vi "DMM_Main.vi"() -> ()   [LabVIEW 2014]
panel:
  out "NumRef":refnum<data-value>
  out "SignalsRef":refnum<data-value>
  in  "Start Process":bool
  in  "Exit Program":bool
  in  "Halt Measuring":bool
  out "Baseline Reference":dbl
  out "Measuring Signals":dbl[](graph)
  in  "Pick Baseline Ref":bool
  out "SampleNum":i32
  out "State":string
  in  "Comments":string
  in  "File Path":path
  in  "Sampling Rate (point / sec)":u32
  in  "Measurement":enum16{"Resistance", "Current"}(ring)
  in  "Baseline Pick":enum16{"Manual", "Auto"}(ring)
  in  "DMM7510 COM":refnum<visa-resource-name>
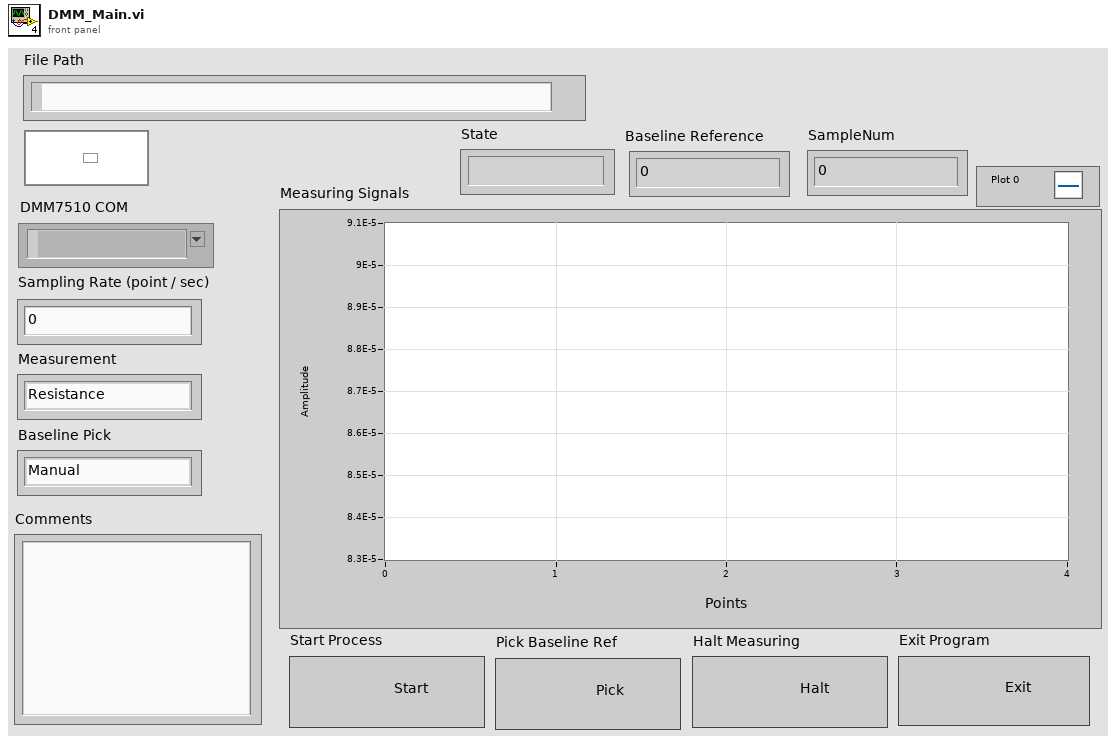
[diagram p1: front panel]
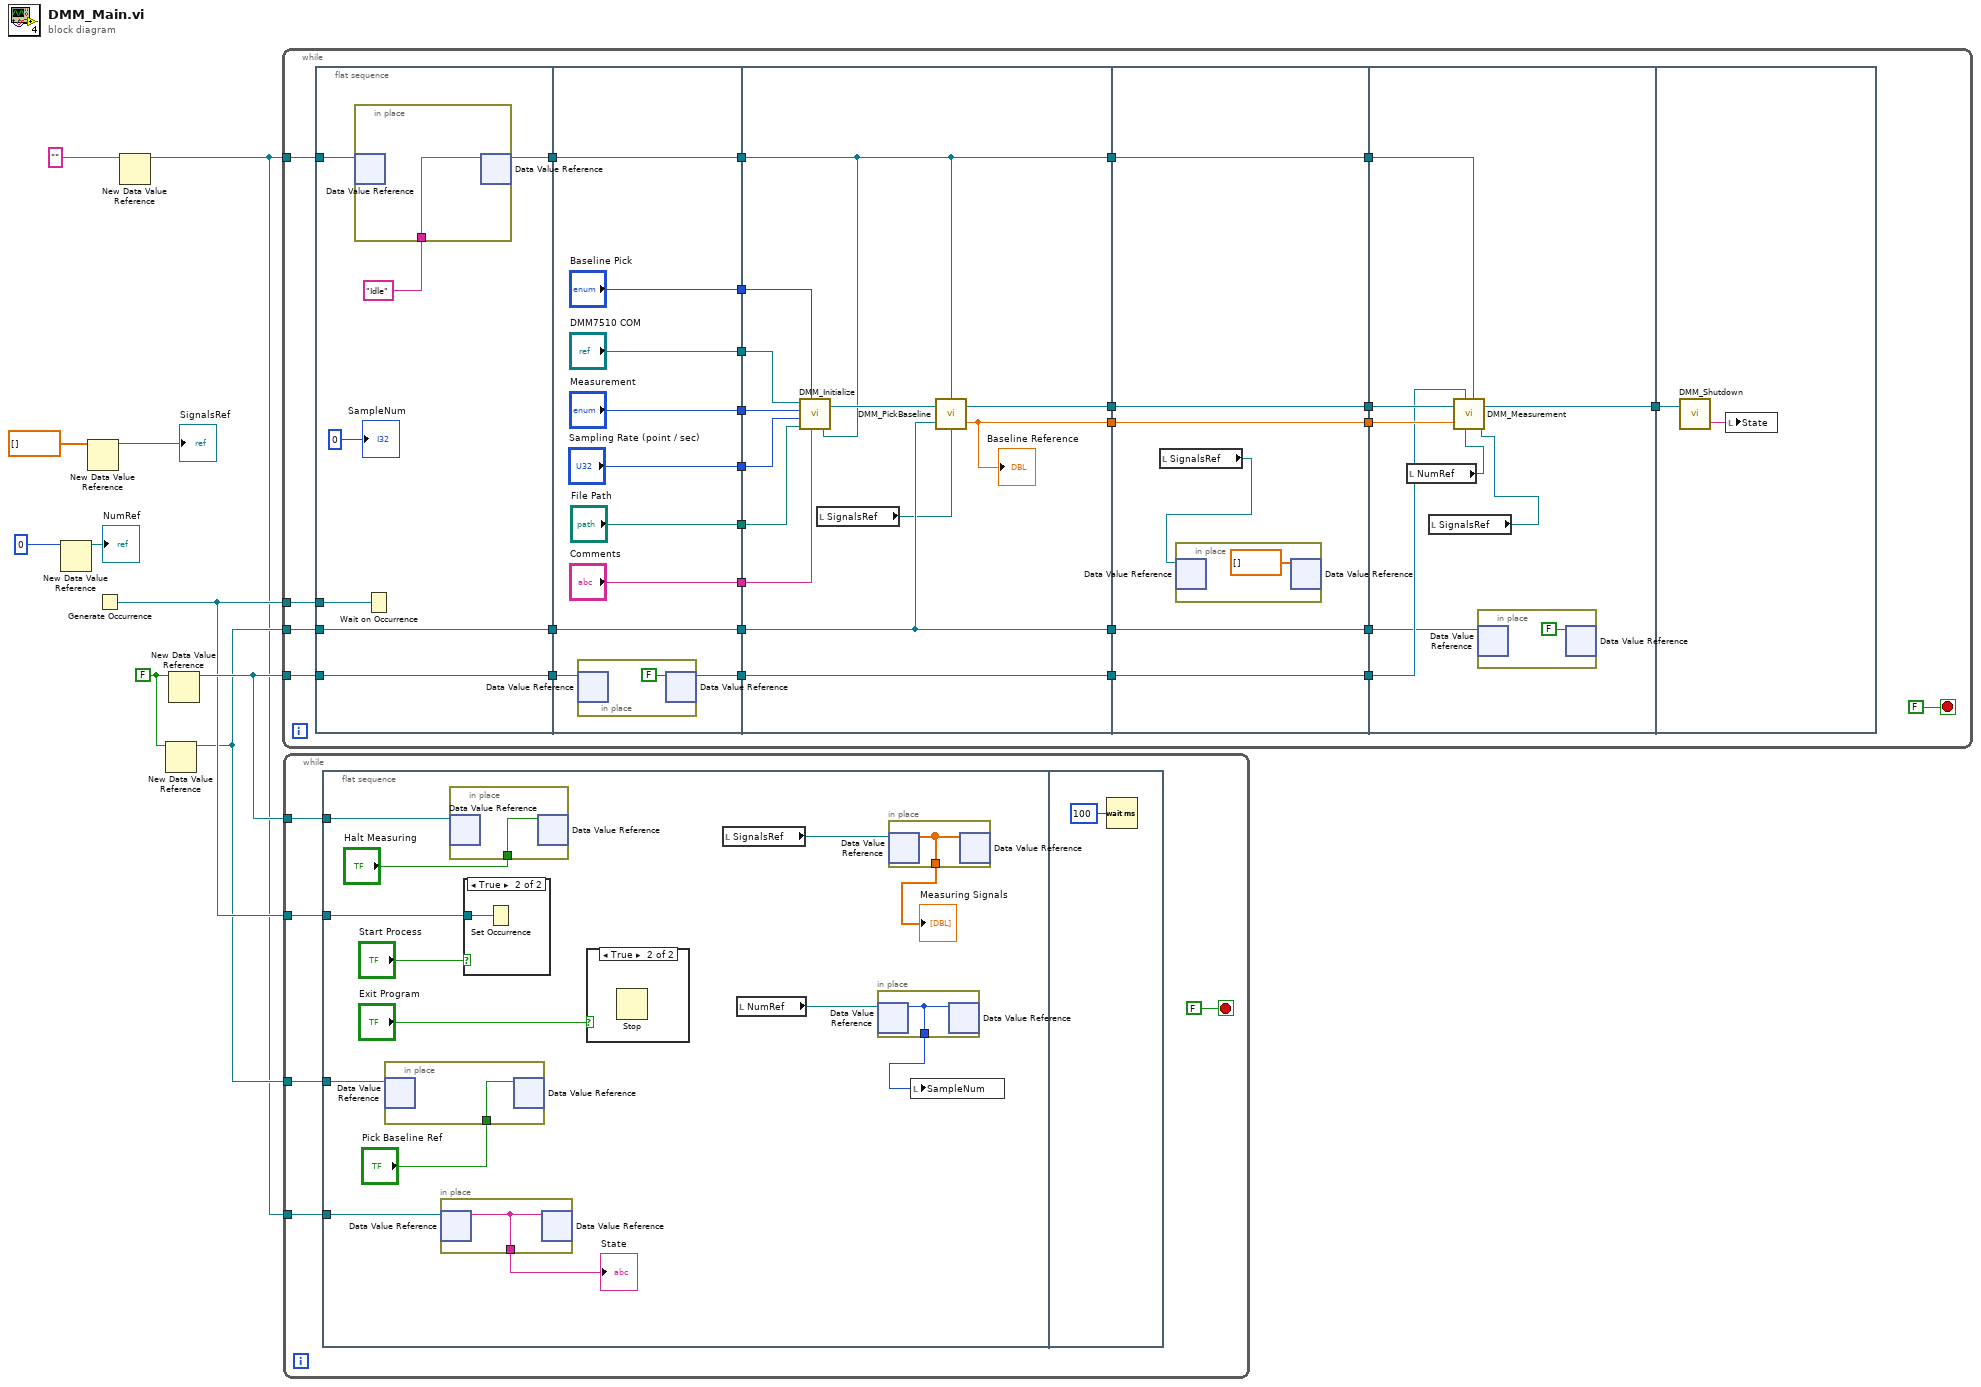
[diagram p0: block diagram]
diagram:
  w8 = FALSE
  n1 = New Data Value Reference(data value=0) -> (data value reference=→"NumRef":refnum<data-value>)  [unwired: 1 in, 1 out]
  n2 = New Data Value Reference(data value=dbl[] []) -> (data value reference=→"SignalsRef":refnum<data-value>)  [unwired: 1 in, 1 out]
  n3 = Generate Occurrence() -> (w9:refnum<k4>)
  n4 = New Data Value Reference(data value="") -> (data value reference=w1:refnum<data-value>)  [unwired: 1 in, 1 out]
  n5 = New Data Value Reference(data value=w8) -> (data value reference=w7:refnum<data-value>)  [unwired: 1 in, 1 out]
  n6 = New Data Value Reference(data value=w8) -> (data value reference=w10:refnum<data-value>)  [unwired: 1 in, 1 out]
  n7 = while {
    tunnel: w10 -> [w30]
    tunnel: w9 -> [w28]
    tunnel: w7 -> [w25]
    tunnel: w1 -> [w15]
    stop <- FALSE stop-if-true
    n8 = flat-sequence {
      tunnel: [w45] -> w31
      tunnel: w30 -> [w45]
      tunnel: w28 -> [w44]
      tunnel: [w42] -> w26
      tunnel: w25 -> [w42]
      tunnel: w15 -> [w41]
      tunnel: [w39] -> w14
      tunnel: ["DMM7510 COM"] -> w38
      tunnel: ["Baseline Pick"] -> w37
      tunnel: ["Measurement"] -> w36
      tunnel: ["Sampling Rate (point / sec)"] -> w35
      tunnel: ["File Path"] -> w34
      tunnel: ["Comments"] -> w33
      tunnel: w31 -> [w50]
      tunnel: [w49] -> w29
      tunnel: w26 -> [w48]
      tunnel: [w48] -> w24
      tunnel: w14 -> [w47]
      tunnel: [w47] -> w13
      tunnel: w38 -> [w70]
      tunnel: w37 -> [w69]
      tunnel: w36 -> [w68]
      tunnel: w35 -> [w67]
      tunnel: w34 -> [w66]
      tunnel: w33 -> [w65]
      tunnel: [w63] -> w23
      tunnel: [w62] -> w21
      tunnel: w29 -> [w61]
      tunnel: [w61] -> w19
      tunnel: w24 -> [w60]
      tunnel: [w60] -> w17
      tunnel: w13 -> [w58]
      tunnel: [w58] -> w11
      tunnel: w23 -> [w76]
      tunnel: [w76] -> w22
      tunnel: w21 -> [w75]
      tunnel: [w75] -> w20
      tunnel: w19 -> [w74]
      tunnel: [w74] -> w18
      tunnel: w17 -> [w73]
      tunnel: [w73] -> w16
      tunnel: [w71] -> w12
      tunnel: w11 -> [w71]
      tunnel: w22 -> [w85]
      tunnel: w20 -> [w84]
      tunnel: w18 -> [w83]
      tunnel: [w82] -> w27
      tunnel: w16 -> [w81]
      tunnel: w12 -> [w78]
      tunnel: w27 -> [w88]
      frame #0 {
        n9 = in-place {
          in-place-border: "Idle" -> [w46]
          n10 = in-place-dvr #1(w41) -> ()  [unwired: 2 out]
          n11 = in-place-dvr #1(w46) -> (w39:refnum<data-value>)  [unwired: 1 out]
        }
        n12 = Wait on Occurrence(2:w44) -> ()  [unwired: 2 in, 1 out]
        "SampleNum" <- 0
      }
      frame #1 {
        n13 = in-place {
          n14 = in-place-dvr #2(w50) -> ()  [unwired: 2 out]
          n15 = in-place-dvr #2(FALSE ("data value")) -> (w49:refnum<data-value>)  [unwired: 1 out]
        }
      }
      frame #2 {
        n16 = call "DMM_Initialize.vi"("StateRef"=w58, "Comments"=w65, "Baseline Pick"=w69, "File Path"=w66, "Sampling Rate (point / sec)"=w67, "Measurement"=w68, "DMM Serial Port"=w70) -> ("Output DMMP"=w64:refnum<class "DMMP.lvclass">)
        n17 = local read "SignalsRef"() -> (w59:refnum<data-value>)
        n18 = call "DMM_PickBaseline.vi"("InputPick"=w60, "SignalRef"=w59, "Input DMMP"=w64, "StateRef"=w58) -> ("Reference"=w62:dbl, "Output DMMP"=w63:refnum<class "DMMP.lvclass">)
        "Baseline Reference" <- w62
      }
      frame #3 {
        n19 = local read "SignalsRef"() -> (w72:refnum<data-value>)
        n20 = in-place {
          n21 = in-place-dvr #3(w72) -> ()  [unwired: 2 out]
          n22 = in-place-dvr #3(dbl[] [] ("data value")) -> ()  [unwired: 2 out]
        }
      }
      frame #4 {
        n23 = local read "NumRef"() -> (w79:refnum<data-value>)
        n24 = local read "SignalsRef"() -> (w80:refnum<data-value>)
        n25 = call "DMM_Measurement.vi"("Reference"=w84, "NumRef"=w79, "SignalRef"=w80, "Input DMMP"=w85, "StopRef"=w83, "StateRef"=w78) -> ("Output DMMP"=w82:refnum<class "DMMP.lvclass">)  [unwired: 1 in]
        n26 = in-place {
          n27 = in-place-dvr #4(w81) -> ()  [unwired: 2 out]
          n28 = in-place-dvr #4(FALSE ("data value")) -> ()  [unwired: 2 out]
        }
      }
      frame #5 {
        n29 = call "DMM_Shutdown.vi"("Input DMMP"=w88) -> ("State"=w87:string)  [unwired: 2 in]
        n30 = local write "State"(w87) -> ()
      }
    }
  }
  n31 = while {
    tunnel: w10 -> [w93]
    tunnel: w9 -> [w92]
    tunnel: w7 -> [w90]
    tunnel: w1 -> [w89]
    stop <- FALSE stop-if-true
    n32 = flat-sequence {
      tunnel: w93 -> [w106]
      tunnel: w92 -> [w103]
      tunnel: w90 -> [w101]
      tunnel: w89 -> [w95]
      frame #0 {
        n33 = in-place {
          in-place-border: "Pick Baseline Ref" -> [w110]
          n34 = in-place-dvr #5(w101) -> ()  [unwired: 2 out]
          n35 = in-place-dvr #5(w110) -> ()  [unwired: 2 out]
        }
        n36 = in-place {
          in-place-border: [w107] -> w94
          n37 = in-place-dvr #6(w95) -> (w107:string)  [unwired: 1 out]
          n38 = in-place-dvr #6(w107) -> ()  [unwired: 2 out]
        }
        "State" <- w94
        n39 = in-place {
          in-place-border: "Halt Measuring" -> [w112]
          n40 = in-place-dvr #7(w106) -> ()  [unwired: 2 out]
          n41 = in-place-dvr #7(w112) -> ()  [unwired: 2 out]
        }
        n42 = case shown="True" "Start Process" {
          tunnel: w103 -> [_ w111]
          frame False {
          }
          frame True {
            n43 = Set Occurrence(w111) -> ()
          }
        }
        n44 = case shown="True" "Exit Program" {
          frame False {
          }
          frame True {
            n45 = Stop() -> ()  [unwired: 1 in]
          }
        }
        n46 = local read "SignalsRef"() -> (w98:refnum<data-value>)
        n47 = local read "NumRef"() -> (w97:refnum<data-value>)
        n48 = in-place {
          in-place-border: [w108] -> w96
          n49 = in-place-dvr #8(w97) -> (w108:i32)  [unwired: 1 out]
          n50 = in-place-dvr #8(w108) -> ()  [unwired: 2 out]
        }
        n51 = in-place {
          in-place-border: [w109] -> w99
          n52 = in-place-dvr #9(w98) -> (w109:dbl[])  [unwired: 1 out]
          n53 = in-place-dvr #9(w109) -> ()  [unwired: 2 out]
        }
        "Measuring Signals" <- w99
        n54 = local write "SampleNum"(w96) -> ()
      }
      frame #1 {
        n55 = Wait (ms)(milliseconds to wait=u32 100) -> ()  [unwired: 1 out]
      }
    }
  }
